vi "AutofocusScan.vi"() -> ()   [LabVIEW 2019]
uses:
  <vilib>/userDefined/High Color/IMAQdx.ctl
  <vilib>/vision/NI_Vision_Development_Module.lvlib
  <vilib>/vision/driver/NI_Vision_Acquisition_Software.lvlib
panel:
  in  "Camera":T1="cam1"
  out "MaxVal":dbl
  out "BestZ":dbl
  out "SDvsZ":string
  out "Sobel_SD":picture
  in  "Z OutputFile":path=path "C:/Users/TTUHEP/Documents/LabVIEW/GantryPrograms/Configs/temp.txt"
  in  "Plot Output File":string="C:\\Users\\TTUHEP\\Documents\\LabVIEW\\GantryPrograms\\LogFiles\\plot.png"
  out "spreadsheet string":string
  out "Image":T2(plugin-control)
  in  "Steps":dbl=20.0
  in  "ScanRange":dbl=0.2
  out "error out":errorcluster
  in  "error in (no error)":errorcluster
  in  "Z":dbl=68.166
  in  "Y":dbl=999.797
  in  "X":dbl=227.948
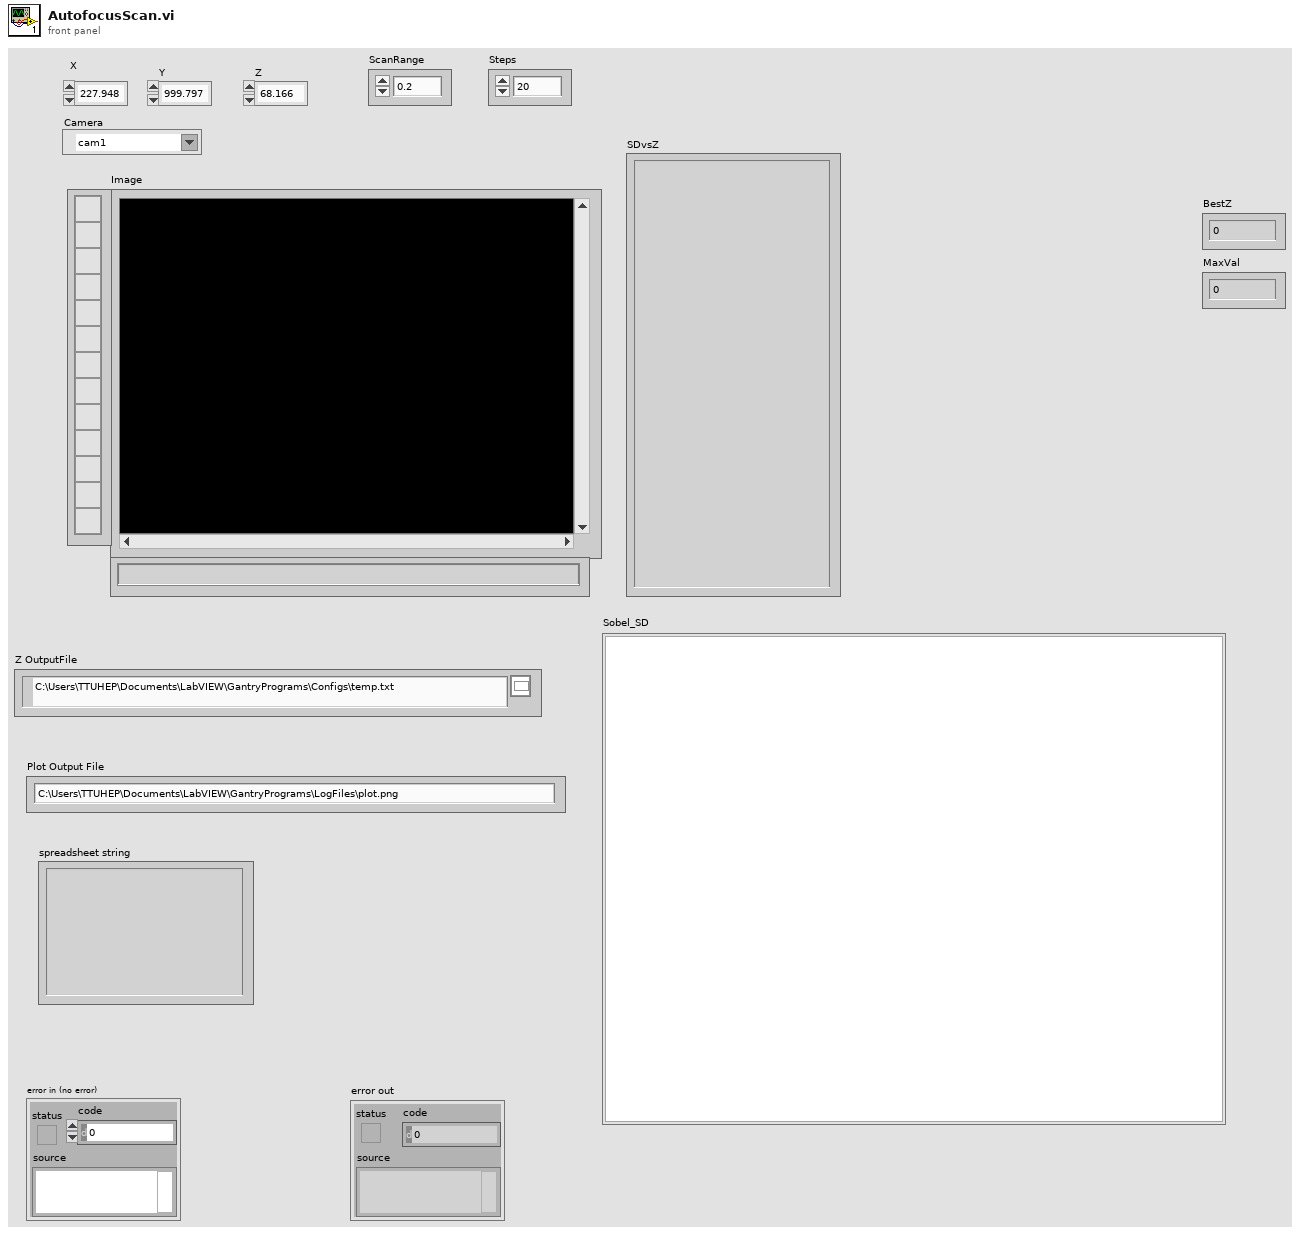
[diagram p1: front panel]
types:
  T1 = typedef "IMAQdx.ctl" = refnum<k21>
  T2 = typedef "IMAQ Image.ctl" = refnum<image>
  T3 = typedef "Image Type" = u32
  T4 = enum16{"open", "replace", "create", "open or create", "replace or create", "replace or create with confirmation"}
  T5 = enum32{"Differentiation", "Gradient", "Prewitt", "Roberts", "Sigma", "Sobel"}
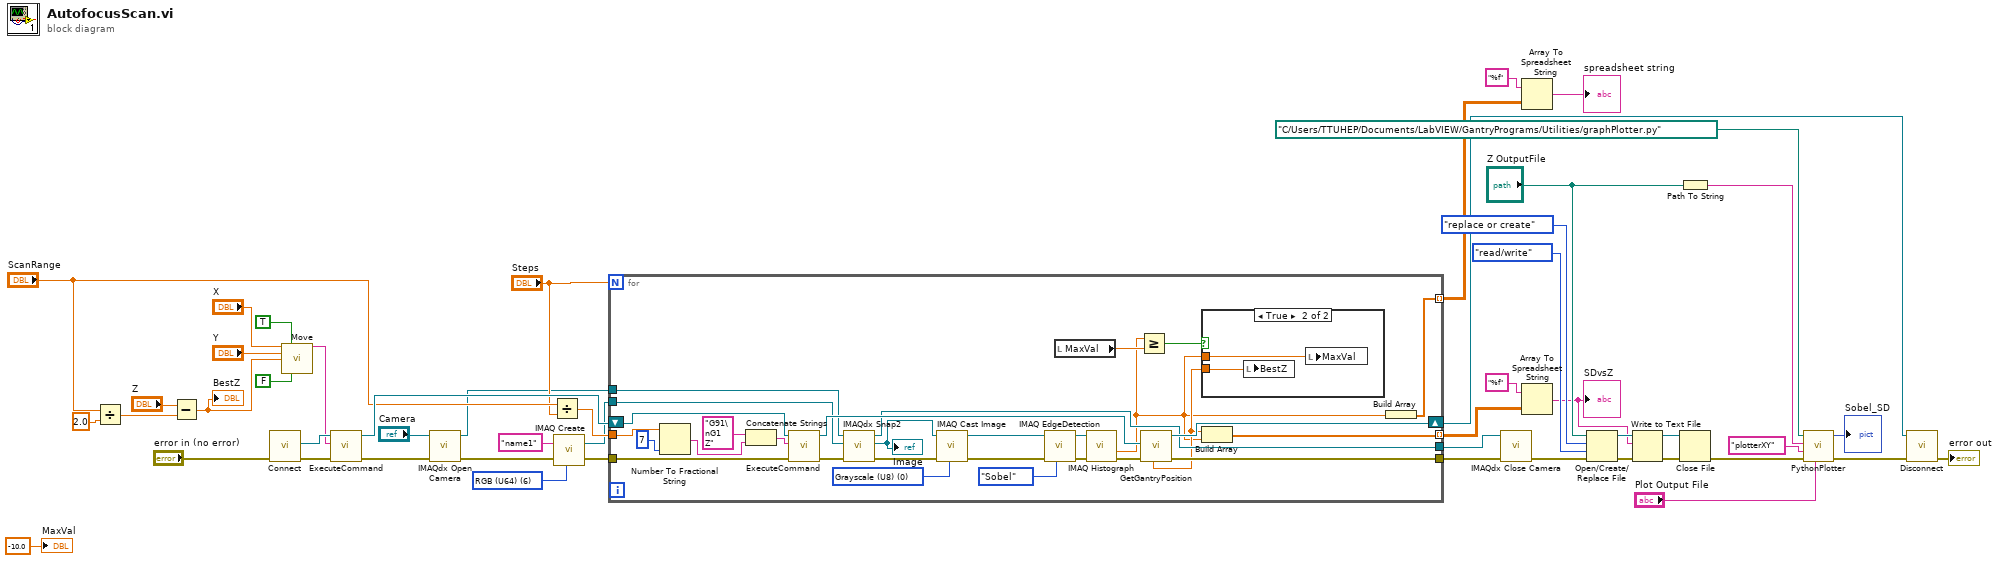
[diagram p0: block diagram]
diagram:
  w10 = T3 6 items=["Grayscale (U8)", "Grayscale (I16)", "Grayscale (SGL)", "Complex (CSG)", "RGB (U32)", "HSL (U32)", "RGB (U64)", "Grayscale (U16)"] ("Image Type")
  n1 = Divide(x="ScanRange", y=2.0) -> (x/y=w48:dbl)
  n2 = Subtract(x="Z", y=w48) -> (x-y=w14:dbl)
  "BestZ" <- w14
  n3 = call "Connect.vi"("error in (no error)"="error in (no error)") -> ("error out"=w3:errorcluster, "controller"=w42:refnum<k24>)  [unwired: 9 in]
  n4 = call "Move.vi"("X"="X", "Absolute"=TRUE, "Y"="Y", "Z"=w14, "Move Z first"=FALSE) -> ("Position Gcode"=w41:string)  [unwired: 10 in]
  n5 = call "ExecuteCommand.vi"("error in (no error)"=w3, "Command Code"=w41, "controller in"=w42) -> ("error out"=w2:errorcluster, "controller out"=w40:refnum<k24>)  [unwired: 6 in, 1 out]
  n6 = call <vilib>:"IMAQdx Open Camera.vi"("error in"=w2, "Session In"="Camera") -> ("error out"=w7:errorcluster, "Session Out"=w8:T1)  [unwired: 8 in]
  n7 = Divide(x="ScanRange", y="Steps") -> (x/y=w37:dbl)
  n8 = call "IMAQ Create"("Image Name"="name1" ("ImageName"), "Image Type"=w10, "error in (no error)"=w7) -> ("New Image"=w9:T2, "error out"=w1:errorcluster)  [unwired: 2 in]
  n9 = for {
    N: "Steps" -> [_]
    tunnel: w1 -> [w67]
    tunnel: w37 -> [w72]
    shift-right: [w62] -> w36
    shift-left: w40 -> [w73]
    tunnel: [w64] -> w5
    tunnel: [w63] -> w21 mode=indexing
    tunnel: [w51] -> w17 mode=indexing
    tunnel: w9 -> [w57]
    tunnel: w8 -> [w59]
    tunnel: [w58] -> w6
    w77 = T3 0 items=["Grayscale (U8)", "Grayscale (I16)", "Grayscale (SGL)", "Complex (CSG)", "RGB (U32)", "HSL (U32)", "RGB (U64)", "Grayscale (U16)"] ("Image Type")
    n10 = Number To Fractional String(number=w72, precision (6)=i16 7) -> (F-format string=w69:string)  [unwired: 2 in]
    n11 = Concatenate Strings("G91\nG1 Z", w69) -> (w68:string)
    n12 = call "ExecuteCommand.vi"("error in (no error)"=w67, "Command Code"=w68, "controller in"=w73) -> ("error out"=w55:errorcluster, "controller out"=w66:refnum<k24>)  [unwired: 6 in, 1 out]
    n13 = call <vilib>:"IMAQdx Snap2.vi"("error in"=w55, "Image In"=w57, "Session In"=w59) -> ("error out"=w54:errorcluster, "Image Out"=w56:T2, "Session Out"=w58:T1)  [unwired: 6 in]
    "Image" <- w56
    n14 = call "IMAQ Cast Image"("Image Type"=w77, "error in (no error)"=w54, "Image Src"=w56) -> ("error out"=w79:errorcluster, "Image Dst Out"=w78:T2)  [unwired: 7 in]
    n15 = call "IMAQ EdgeDetection"("Method"=T5."Sobel", "error in (no error)"=w79, "Image Src"=w78) -> ("error out"=w76:errorcluster, "Image Dst Out"=w75:T2)  [unwired: 7 in]
    n16 = local read "MaxVal"() -> (w61:dbl)
    n17 = call "IMAQ Histograph"("error in (no error)"=w76, "Image"=w75) -> ("error out"=w65:errorcluster, "Standard  Deviation"=w52:sgl)  [unwired: 6 in, 2 out]
    n18 = Greater Or Equal?(x=w52, y=w61) -> (x >= y?=w60:bool)
    n19 = call "GetGantryPosition.vi"("error in (no error)"=w65, "Controller In"=w66) -> ("error out"=w64:errorcluster, "controller out"=w62:refnum<k24>, "Position Z"=w53:dbl)  [unwired: 3 in, 4 out]
    n20 = case shown="True" w60 {
      tunnel: w52 -> [_ w81]
      tunnel: w53 -> [_ w80]
      frame False {
      }
      frame True {
        n21 = local write "BestZ"(w80) -> ()
        n22 = local write "MaxVal"(w81) -> ()
      }
    }
    n23 = Build Array(w53, w52) -> (w51:dbl[])
    n24 = Build Array(w52) -> (w63:sgl[])
  }
  n25 = call <vilib>:"IMAQdx Close Camera.vi"("error in"=w5, "Session In"=w6) -> ("error out"=w4:errorcluster)  [unwired: 9 in]
  n26 = Array To Spreadsheet String(array=w21, 3:"%f" ("format string")) -> (spreadsheet string=→"spreadsheet string":string)  [unwired: 1 in]
  n27 = Array To Spreadsheet String(array=w17, 3:"%f" ("format string")) -> (spreadsheet string=w15:string)  [unwired: 1 in]
  "SDvsZ" <- w15
  n28 = Open/Create/Replace File(file path (use dialog)="Z OutputFile", error in=w4, operation (0:open)=T4."replace or create", access (0:read/write)=enum16{"read/write", "read-only", "write-only"}."read/write") -> (refnum out=w29:refnum<file>, error out=w30:errorcluster)  [unwired: 2 in, 1 out]
  n29 = Write to Text File(file (use dialog)=w29, text=w15, error in=w30) -> (refnum out=w32:refnum<file>, error out=w31:errorcluster)  [unwired: 1 in, 1 out]
  n30 = Path To String(path="Z OutputFile") -> (string=w24:string)
  n31 = Close File(refnum=w32, error in=w31) -> (error out=w23:errorcluster)  [unwired: 1 out]
  n32 = call "PythonPlotter.vi"("Output File"="Plot Output File", "error in (no error)"=w23, "Function Name"="plotterXY", "Input File"=w24, "Python Path"=path "C:/Users/TTUHEP/Documents/LabVIEW/GantryPrograms/Utilities/graphPlotter.py") -> ("error out"=w19:errorcluster, "HighVSPosition"=→"Sobel_SD":picture)  [unwired: 4 in]
  n33 = call "Disconnect.vi"("error in (no error)"=w19, "controller"=w36) -> ("error out"=→"error out":errorcluster)  [unwired: 9 in]
  "MaxVal" <- -10.0 ("MaxVal")
